vi "Boolean to Double Solenoid.vi"(5 "Invert? (F)":bool, 11 "Dir?":bool) -> (3 "Value":T1)   [LabVIEW 2016, in "Intake.lvlib"]
uses:
  SubSystems/Intake/Intake.lvlib
  <vilib>/Rock Robotics/WPI/Solenoid/WPI_SolenoidValue.ctl
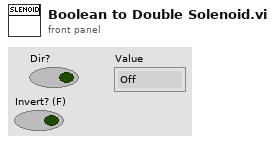
[diagram p1: front panel]
types:
  T1 = typedef "WPI_SolenoidValue.ctl" = enum16{"Off", "On", "Forward", "Reverse"}
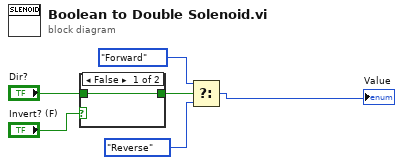
[diagram p0: block diagram]
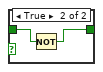
[diagram p2: hidden frame]
diagram:
  n1 = case shown="False" "Invert? (F)" {
    tunnel: "Dir?" -> [w7 w9]
    tunnel: [w7 w8] -> w2
    frame False {
    }
    frame True {
      n2 = Not(x=w9) -> (.not. x?=w8:bool)
    }
  }
  n3 = Select(t=WPI_SolenoidValue."Forward" ("Value"), s=w2, f=WPI_SolenoidValue."Reverse" ("Value")) -> (s? t:f=→"Value":T1)
